vi "translate_digital_outputs.vi"(0 "simple_actions":T3, 2 "do_value (in)":u32, 3 "digital_output_items (in)":T1[](array[typedef])) -> (16 "do_value (out)":u32, 17 "digital_output_items (out)":T1[](array[typedef]))   [LabVIEW 2012]
doc: "Translates the digital output values TO and FROM the numeric value interpretted by the API call.\n\nProduced By:\n\nChristopher Lemieux\nKod Integrations, LLC\n4835 Marianne Drive\nMount Airy, MD 21771\nhttp://www.kodintegrations.com\nemail: clemieux@kodintegrations.com\nphone: (240) 687-1288"
uses:
  controls/simple_actions.ctl
  controls/digital_output_item_group.ctl
  controls/digital_output_items.ctl
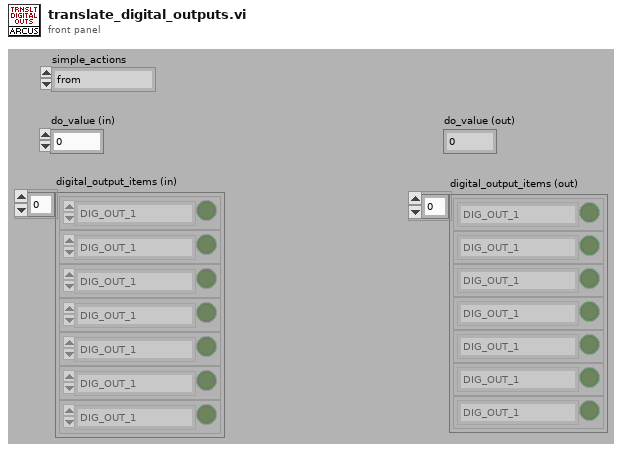
[diagram p1: front panel]
types:
  T1 = typedef "digital_output_item_group.ctl" = cluster{"item":T2, "status":bool}
  T2 = typedef "digital_output_items.ctl" = enum16{"DIG_OUT_1", "DIG_OUT_2"}
  T3 = typedef "simple_actions.ctl" = enum16{"from", "to"}
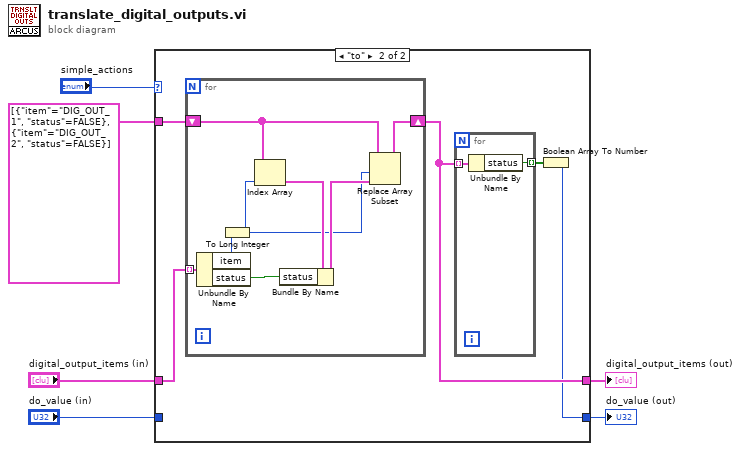
[diagram p0: block diagram]
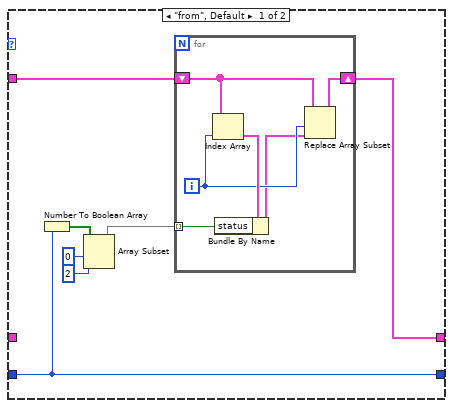
[diagram p2: hidden frame]
diagram:
  n1 = case shown="\"to\"" "simple_actions" {
    tunnel: "do_value (in)" -> [w7 _]
    tunnel: [w9 w22] -> w4
    tunnel: T1[] [{"item"=enum."DIG_OUT_1", "status"=FALSE}, {"item"=enum."DIG_OUT_2", "status"=FALSE}] ("polarity_items (in)") -> [w8 w24]
    tunnel: "digital_output_items (in)" -> [_ w23]
    tunnel: [w7 w20] -> w1
    frame "from", Default {
      n2 = Number To Boolean Array(number=w7) -> (Boolean array=w13:bool[])
      n3 = Array Subset(array=w13, index=0, length=2) -> (w10:bool[])
      n4 = for {
        shift-right: [w14] -> w9
        shift-left: w8 -> [w17]
        tunnel: w10 -> [w18] mode=indexing
        i -> [w16]
        n5 = Index Array(array=w17, index=w16) -> (element=w19:T1)
        n6 = Bundle By Name(cluster=w19, "status"=w18) -> (w15:T1)
        n7 = Replace Array Subset(array=w17, new element=w15, index=w16) -> (w14:T1[])
      }
    }
    frame "to" {
      n8 = for {
        shift-right: [w28] -> w22
        shift-left: w24 -> [w27]
        tunnel: w23 -> [w32] mode=indexing
        n9 = Unbundle By Name(w32) -> ("item"=w31:T2, "status"=w30:bool)
        n10 = To Long Integer(number=w31) -> (32bit integer=w29:i32)
        n11 = Index Array(array=w27, index=w29) -> (element=w33:T1)
        n12 = Bundle By Name(cluster=w33, "status"=w30) -> (w34:T1)
        n13 = Replace Array Subset(array=w27, new element=w34, index=w29) -> (w28:T1[])
      }
      n14 = for {
        tunnel: w22 -> [w26] mode=indexing
        tunnel: [w25] -> w21 mode=indexing
        n15 = Unbundle By Name(w26) -> ("status"=w25:bool)
      }
      n16 = Boolean Array To Number(Boolean array=w21) -> (number=w20:u32)
    }
  }
  "digital_output_items (out)" <- w4
  "do_value (out)" <- w1
